vi "DeleteActionToRemainList.vi"(8 "error in (no error)":errorcluster, 9 "ManualFlg":bool, 10 "Remaining Action":refnum<vi>, 11 "Main Class in":refnum<class "Main Class.lvclass">) -> (0 "error out":errorcluster, 3 "Main Class out":refnum<class "Main Class.lvclass">)   [LabVIEW 2019, in "Main Class.lvclass"]
uses:
  Main Class.lvclass
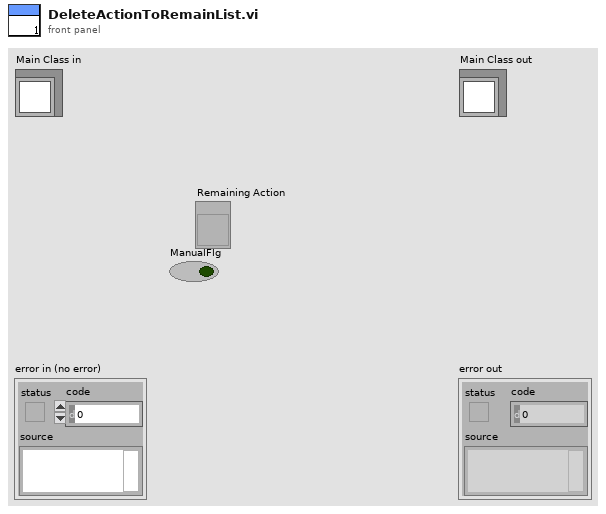
[diagram p1: front panel]
types:
  T1 = enum16{"Initial", "Add", "Read", "Delete & Check"}
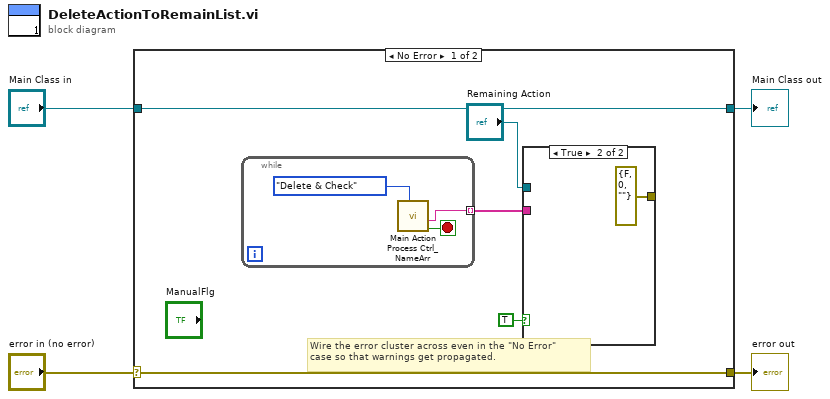
[diagram p0: block diagram]
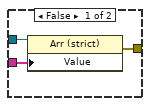
[diagram p2: hidden frame]
diagram:
  n1 = case shown="No Error" "error in (no error)" {
    selector: "error in (no error)" -> [w8 w18]
    tunnel: [w8 w18] -> w3
    tunnel: [w9 w17] -> w1
    tunnel: "Main Class in" -> [w9 w17]
    frame No Error {
      # "Wire the error cluster across even in the \"No Error\"\ncase so that warnings get propagated."
      n2 = while {
        tunnel: [w14] -> w7 mode=indexing
        stop <- w15 stop-if-true
        n3 = call "Main Action Process Ctrl_NameArr.vi"("Action"=T1."Delete & Check") -> ("Finish"=w15:bool, "Delete Action"=w14:string)  [unwired: 6 in, 3 out]
      }
      n4 = case shown="True" TRUE {
        tunnel: "Remaining Action" -> [w12 _]
        tunnel: w7 -> [w11 _]
        tunnel: [w10 errorcluster {"status"=FALSE, "code"=0, "source"=""} ("error out")] -> _
        frame False {
          n5 = property class="Arr (strict)"(reference=w12, "Value"=w11) -> (error out=w10:errorcluster)  [unwired: 1 in, 1 out]
        }
        frame True {
        }
      }
    }
    frame Error {
    }
  }
  "error out" <- w3
  "Main Class out" <- w1
